vi "ReadSizeMat_1DArray-2DPoint-I32.vi"(8 "error in":errorcluster, 11 "Array in":T1[](array[typedef])) -> (0 "error out":errorcluster, 1 "Height":i32, 2 "Width":i32, 3 "Array out":T1[](array[typedef]), 4 "Channel":i32)   [LabVIEW 2020, in "OpenLvVision_OpenCv.lvlib"]
doc: "Read size of the datatype\nNo malleable to breake vi inlining!"
uses:
  OpenLvVision_OpenCv.lvlib
  TypeDef/Point/2D_PointI32.ctl
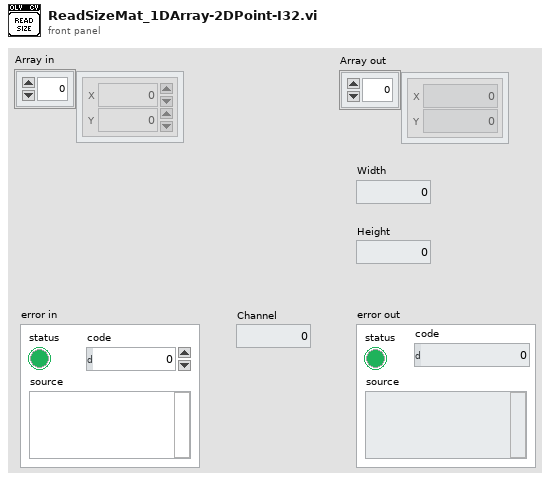
[diagram p1: front panel]
types:
  T1 = typedef "OpenLvVision_OpenCv.lvlib/2D_PointI32.ctl" = cluster{"X":i32, "Y":i32}
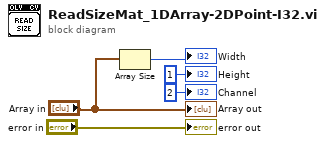
[diagram p0: block diagram]
diagram:
  n1 = Array Size(array="Array in") -> (size(s)=→"Width":i32)
  "error out" <- "error in"
  "Height" <- 1 ("Height")
  "Channel" <- 2 ("Channel")
  "Array out" <- "Array in"
